vi "Render.vi"(8 "error in (no error)":errorcluster, 11 "Game in":refnum<class "Game.lvclass">) -> (0 "error out":errorcluster, 3 "Game out":refnum<class "Game.lvclass">)   [LabVIEW 2019, in "RT_Game.lvlib" / "Game.lvclass"]
uses:
  Game.lvclass
  Game.lvclass/Game.ctl
  RT_Sprite/RT_Sprite.lvclass
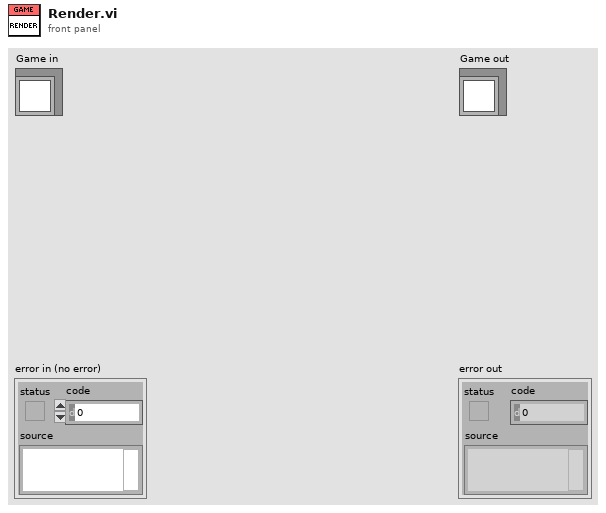
[diagram p1: front panel]
types:
  T1 = typedef "RT_Game.lvlib/Game.lvclass/SpritesCluster.ctl" = cluster{"Sprite1":refnum<class "RT_Sprite.lvclass">, "Sprite2":refnum<class "RT_Sprite.lvclass">, "Sprite3":refnum<class "RT_Sprite.lvclass">}
  T2 = cluster{"Sprites out[0]":refnum<class "RT_Sprite.lvclass">, "Sprites out[1]":refnum<class "RT_Sprite.lvclass">, "Sprites out[2]":refnum<class "RT_Sprite.lvclass">}
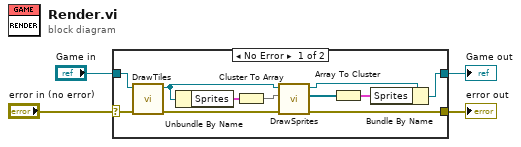
[diagram p0: block diagram]
diagram:
  n1 = case shown="No Error" "error in (no error)" {
    selector: "error in (no error)" -> [w15 w17]
    tunnel: [w12 w17] -> w3
    tunnel: [w13 w16] -> w1
    tunnel: "Game in" -> [w9 w16]
    frame No Error {
      n2 = call "DrawTiles.vi"("error in (no error)"=w15, "Game in"=w9) -> ("error out"=w14:errorcluster, "Game out"=w7:refnum<class "Game.lvclass">)  [unwired: 8 in]
      n3 = Unbundle By Name(w7) -> ("Sprites"=w11:T1)
      n4 = Cluster To Array(cluster=w11) -> (array=w6:refnum<class "RT_Sprite.lvclass">[])
      n5 = call "DrawSprites.vi"("error in (no error)"=w14, "Sprites in"=w6, "Game in"=w7) -> ("error out"=w12:errorcluster, "Sprites out"=w10:refnum<class "RT_Sprite.lvclass">[], "Game out"=w8:refnum<class "Game.lvclass">)  [unwired: 6 in]
      n6 = Array To Cluster(array=w10) -> (cluster=w5:T2)
      n7 = Bundle By Name(cluster=w8, "Sprites"=w5) -> (w13:refnum<class "Game.lvclass">)
    }
    frame Error {
    }
  }
  "error out" <- w3
  "Game out" <- w1
